vi "test-TimeInterpRotation-Test1.vi"() -> (3 "All tests passed":bool)   [LabVIEW 2019]
uses:
  <vilib>/Rock Robotics/WPI/ThirdParty/JAS_Junk/TrajLib/ROTATION2D.ctl
  <vilib>/Rock Robotics/WPI/ThirdParty/JAS_Junk/TrajLib/Util_CalcDist.vi
  <vilib>/Rock Robotics/WPI/ThirdParty/JAS_Junk/TrajLib/TimeInterpRotation2d_CleanUp.vi
  <vilib>/gmath/interp.llb/Search Ordered Table.vi
  <vilib>/Rock Robotics/WPI/ThirdParty/JAS_Junk/TrajLib/Trajectory_Library.lvlib
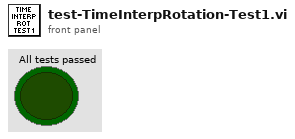
[diagram p1: front panel]
types:
  T1 = typedef "Trajectory_Library.lvlib/ROTATION2D.ctl" = cluster{"VALUE":dbl, "COS":dbl, "SIN":dbl}
  T2 = typedef "Trajectory_Library.lvlib/TIME_INTERPOLATABLE_ROTATION.ctl" = cluster{"TimeStamps":dbl[], "RotationValues":T1[], "Min_TimeStamp":dbl, "Max_TimeStamp":dbl, "ItemCount":i32, "MaxBufferTime":dbl}
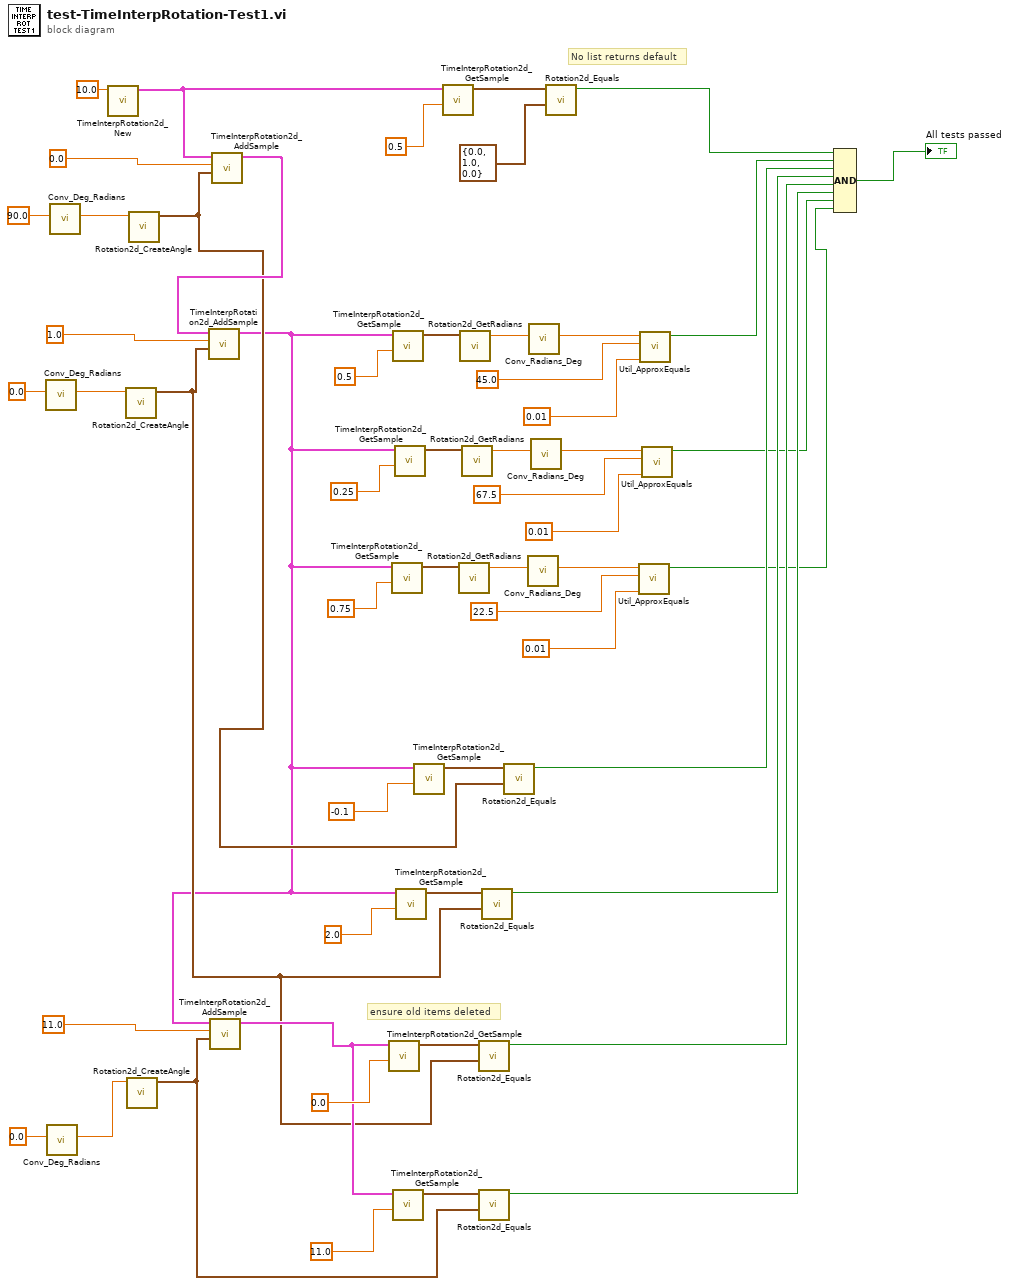
[diagram p0: block diagram]
diagram:
  # "ensure old items deleted"
  # "No list returns default"
  n1 = call <vilib>:"Conv_Deg_Radians.vi"("Degress"=0.0) -> ("Radians"=w21:dbl)  [unwired: 10 in]
  n2 = call <vilib>:"Conv_Deg_Radians.vi"("Degress"=0.0) -> ("Radians"=w22:dbl)  [unwired: 10 in]
  n3 = call <vilib>:"Conv_Deg_Radians.vi"("Degress"=90.0) -> ("Radians"=w20:dbl)  [unwired: 10 in]
  n4 = call <vilib>:"TimeInterpRotation2d_New.vi"("MaxTime"=10.0) -> ("TimeInterpRotation"=w41:T2)  [unwired: 10 in]
  n5 = call <vilib>:"Rotation2d_CreateAngle.vi"("Angle"=w21) -> ("ROTATION"=w23:T1)  [unwired: 10 in]
  n6 = call <vilib>:"Rotation2d_CreateAngle.vi"("Angle"=w22) -> ("ROTATION"=w26:T1)  [unwired: 10 in]
  n7 = call <vilib>:"Rotation2d_CreateAngle.vi"("Angle"=w20) -> ("ROTATION"=w19:T1)  [unwired: 10 in]
  n8 = call <vilib>:"TimeInterpRotation2d_AddSample.vi"("RotationValue"=w19, "TimeStamp"=0.0, "in TimeInterpRotation"=w41) -> ("out TimeInterpRotation"=w43:T2)  [unwired: 7 in, 1 out]
  n9 = call <vilib>:"TimeInterpRotation2d_AddSample.vi"("RotationValue"=w23, "TimeStamp"=1.0, "in TimeInterpRotation"=w43) -> ("out TimeInterpRotation"=w3:T2)  [unwired: 7 in, 1 out]
  n10 = call <vilib>:"TimeInterpRotation2d_AddSample.vi"("RotationValue"=w26, "TimeStamp"=11.0, "in TimeInterpRotation"=w3) -> ("out TimeInterpRotation"=w27:T2)  [unwired: 7 in, 1 out]
  n11 = call <vilib>:"TimeInterpRotation2d_GetSample.vi"("TimeStamp"=0.0, "TimeInterpRotation"=w27) -> ("OutputRotation"=w30:T1)  [unwired: 9 in]
  n12 = call <vilib>:"TimeInterpRotation2d_GetSample.vi"("TimeStamp"=0.75, "TimeInterpRotation"=w3) -> ("OutputRotation"=w5:T1)  [unwired: 9 in]
  n13 = call <vilib>:"TimeInterpRotation2d_GetSample.vi"("TimeStamp"=0.5, "TimeInterpRotation"=w3) -> ("OutputRotation"=w18:T1)  [unwired: 9 in]
  n14 = call <vilib>:"TimeInterpRotation2d_GetSample.vi"("TimeStamp"=11.0, "TimeInterpRotation"=w27) -> ("OutputRotation"=w28:T1)  [unwired: 9 in]
  n15 = call <vilib>:"TimeInterpRotation2d_GetSample.vi"("TimeStamp"=0.25, "TimeInterpRotation"=w3) -> ("OutputRotation"=w11:T1)  [unwired: 9 in]
  n16 = call <vilib>:"TimeInterpRotation2d_GetSample.vi"("TimeStamp"=2.0, "TimeInterpRotation"=w3) -> ("OutputRotation"=w36:T1)  [unwired: 9 in]
  n17 = call <vilib>:"TimeInterpRotation2d_GetSample.vi"("TimeStamp"=-0.1, "TimeInterpRotation"=w3) -> ("OutputRotation"=w38:T1)  [unwired: 9 in]
  n18 = call <vilib>:"TimeInterpRotation2d_GetSample.vi"("TimeStamp"=0.5, "TimeInterpRotation"=w41) -> ("OutputRotation"=w42:T1)  [unwired: 9 in]
  n19 = call <vilib>:"Rotation2d_GetRadians.vi"("in ROTATION"=w5) -> ("AngleRadians"=w4:dbl)  [unwired: 10 in]
  n20 = call <vilib>:"Rotation2d_GetRadians.vi"("in ROTATION"=w18) -> ("AngleRadians"=w17:dbl)  [unwired: 10 in]
  n21 = call <vilib>:"Rotation2d_GetRadians.vi"("in ROTATION"=w11) -> ("AngleRadians"=w10:dbl)  [unwired: 10 in]
  n22 = call <vilib>:"Rotation2d_Equals.vi"("other ROTATION"=w23, "in ROTATION"=w30) -> ("Equals"=w25:bool)  [unwired: 9 in]
  n23 = call <vilib>:"Rotation2d_Equals.vi"("other ROTATION"=w26, "in ROTATION"=w28) -> ("Equals"=w24:bool)  [unwired: 9 in]
  n24 = call <vilib>:"Rotation2d_Equals.vi"("other ROTATION"=w23, "in ROTATION"=w36) -> ("Equals"=w34:bool)  [unwired: 9 in]
  n25 = call <vilib>:"Rotation2d_Equals.vi"("other ROTATION"=w19, "in ROTATION"=w38) -> ("Equals"=w35:bool)  [unwired: 9 in]
  n26 = call <vilib>:"Conv_Radians_Deg.vi"("Radians"=w4) -> ("Degrees"=w8:dbl)  [unwired: 10 in]
  n27 = call <vilib>:"Conv_Radians_Deg.vi"("Radians"=w17) -> ("Degrees"=w48:dbl)  [unwired: 10 in]
  n28 = call <vilib>:"Conv_Radians_Deg.vi"("Radians"=w10) -> ("Degrees"=w14:dbl)  [unwired: 10 in]
  n29 = call <vilib>:"Rotation2d_Equals.vi"("other ROTATION"=T1 {"VALUE"=0.0, "COS"=1.0, "SIN"=0.0} ("ROTATION"), "in ROTATION"=w42) -> ("Equals"=w16:bool)  [unwired: 9 in]
  n30 = call <vilib>:"Util_ApproxEquals.vi"("Tolerance"=0.01, "Value 2"=22.5, "Value 1"=w8) -> ("ApproxEquals"=w1:bool)  [unwired: 8 in]
  n31 = call <vilib>:"Util_ApproxEquals.vi"("Tolerance"=0.01, "Value 2"=45.0, "Value 1"=w48) -> ("ApproxEquals"=w45:bool)  [unwired: 8 in]
  n32 = call <vilib>:"Util_ApproxEquals.vi"("Tolerance"=0.01, "Value 2"=67.5, "Value 1"=w14) -> ("ApproxEquals"=w2:bool)  [unwired: 8 in]
  n33 = Compound Arithmetic op=AND(w16, w45, w35, w34, w25, w24, w2, w1) -> (→"All tests passed":bool)
